vi "log_logger.vi"() -> ()   [LabVIEW 2012]
panel:
  out "Log open":bool
  out "Event count":dbl
  in  "Stop":bool
  in  "Start":bool
  in  "Log file":path
  in  "stop":bool
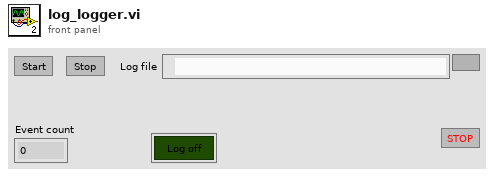
[diagram p1: front panel]
types:
  T1 = enum16{"open", "replace", "create", "open or create", "replace or create", "replace or create with confirmation"}
  T2 = typedef "log_event.ctl" = cluster{"Facility ID":i32, "Severity":enum16{"OK", "Debug", "Warn", "Error"}, "Timestamp":timestamp, "Facility":string, "State":string, "Message":string}
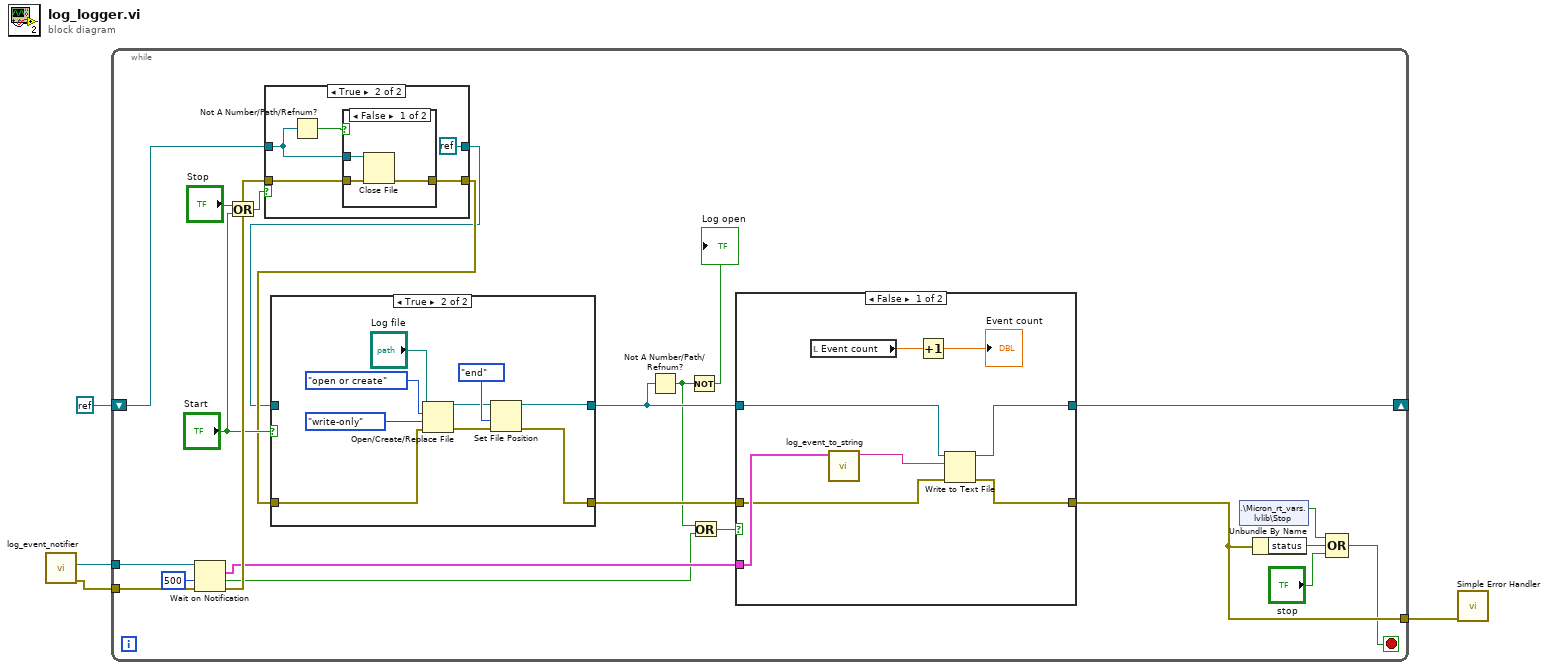
[diagram p0: block diagram]
diagram:
  n1 = call "log_event_notifier.vi"() -> ("error out"=w2:errorcluster, "Log event notifier"=w4:refnum<notifier>)  [unwired: 10 in]
  n2 = while {
    tunnel: w4 -> [w27]
    tunnel: [w26] -> w3
    tunnel: w2 -> [w25]
    shift-right: [w8] -> _
    shift-left: refnum<k0> refnum -> [w9]
    stop <- w7 stop-if-true
    n3 = Wait on Notification(notifier=w27, timeout in ms (-1)=500, error in (no error)=w25) -> (notification=w15:T2, timed out?=w11:bool, error out=w20:errorcluster)  [unwired: 1 in, 1 out]
    n4 = Or(x="Stop", y="Start") -> (x .or. y?=w18:bool)
    n5 = case shown="True" w18 {
      tunnel: w9 -> [w29 w32]
      tunnel: w20 -> [w28 w34]
      tunnel: [w28 w33] -> w16
      tunnel: [w29 refnum<k0> refnum] -> w13
      frame False {
      }
      frame True {
        n6 = Not A Number/Path/Refnum?(number/path/refnum=w32) -> (NaN/Path/Refnum?=w31:bool)
        n7 = case shown="False" w31 {
          tunnel: w34 -> [w37 w38]
          tunnel: [w36 w38] -> w33
          tunnel: w32 -> [w35 _]
          frame False {
            n8 = Close File(refnum=w35, error in=w37) -> (error out=w36:errorcluster)  [unwired: 1 out]
          }
          frame True {
          }
        }
      }
    }
    n9 = case shown="True" "Start" {
      tunnel: [w40 w42] -> w12
      tunnel: w16 -> [w39 w46]
      tunnel: [w39 w41] -> w14
      tunnel: w13 -> [w40 _]
      frame False {
      }
      frame True {
        n10 = Open/Create/Replace File(file path (use dialog)="Log file", error in=w46, operation (0:open)=T1."open or create", access (0:read/write)=enum16{"read/write", "read-only", "write-only"}."write-only") -> (refnum out=w43:refnum<file>, error out=w45:errorcluster)  [unwired: 2 in, 1 out]
        n11 = Set File Position(refnum=w43, from (0:start)=enum16{"start", "end", "current"}."end", error in=w45) -> (refnum out=w42:refnum<file>, error out=w41:errorcluster)  [unwired: 1 in]
      }
    }
    n12 = Not A Number/Path/Refnum?(number/path/refnum=w12) -> (NaN/Path/Refnum?=w5:bool)
    n13 = Not(x=w5) -> (.not. x?=→"Log open":bool)
    n14 = Or(x=w5, y=w11) -> (x .or. y?=w10:bool)
    n15 = case shown="False" w10 {
      tunnel: w12 -> [w55 w59]
      tunnel: [w54 w59] -> w8
      tunnel: w15 -> [w56 _]
      tunnel: w14 -> [w53 w58]
      tunnel: [w52 w58] -> w26
      frame False {
        n16 = local read "Event count"() -> (w51:dbl)
        n17 = call "log_event_to_string.vi"("Log event"=w56) -> ("String"=w57:string)  [unwired: 10 in]
        n18 = Increment(x=w51) -> (x+1=→"Event count":dbl)
        n19 = Write to Text File(file (use dialog)=w55, text=w57, error in=w53) -> (refnum out=w54:refnum<file>, error out=w52:errorcluster)  [unwired: 1 in, 1 out]
      }
      frame True {
      }
    }
    n20 = shared-variable ".\\Micron_rt_vars.lvlib\\Stop"() -> (w23:bool)  [unwired: 1 in, 1 out]
    n21 = Unbundle By Name(w26) -> ("status"=w22:bool)
    n22 = Compound Arithmetic op=OR(w23, w22, "stop") -> (w7:bool)
  }
  n23 = call <vilib>:"Simple Error Handler.vi"("error in (no error)"=w3) -> ()  [unwired: 4 in, 5 out]
